vi "Controller 2.vi"(0 "Joystick Multiplier":dbl=1.0) -> (1 "Axes":T1, 2 "Buttons":T2)   [LabVIEW 2013]
uses:
  <vilib>/Rock Robotics/WPI/Joystick/WPI_JoystickGetSetRefNum.vi
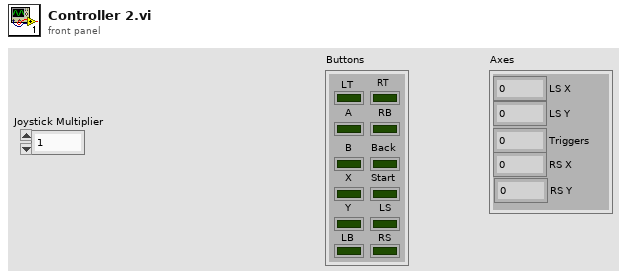
[diagram p1: front panel]
types:
  T1 = cluster{"LS X":dbl, "LS Y":dbl, "Triggers":dbl, "RS X":dbl, "RS Y":dbl}
  T2 = cluster{"LT":bool, "RT":bool, "A":bool, "B":bool, "X":bool, "Y":bool, "LB":bool, "RB":bool, "Back":bool, "Start":bool, "LS":bool, "RS":bool}
  T3 = typedef "WPI_JoystickDevRef.ctl" = cluster{"Device":T4}
  T4 = typedef "WPI_JoystickDeviceEnum.ctl" = enum16{"USB 1", "USB 2", "USB 3", "USB 4", "Kinect 1", "Kinect 2"}
  T5 = typedef "WPI_JoystickButtonState.ctl" = cluster{"Button 1":bool, "Button 2":bool, "Button 3":bool, "Button 4":bool, "Button 5":bool, "Button 6":bool, "Button 7":bool, "Button 8":bool, "Button 9":bool, "Button 10":bool, "Button 11":bool, "Button 12":bool}
  T6 = cluster{"axis 1 (x)":dbl, "axis 2 (y)":dbl, "axis 3 (throttle)":dbl, "axis 4":dbl, "axis 5":dbl, "axis 6":dbl}
  T7 = cluster{"axis 1 (x)":dbl, "axis 2 (y)":dbl, "axis 3 (throttle)":dbl, "axis 4":dbl, "axis 5":dbl}
  T8 = cluster{bool, bool, "Button 1":bool, "Button 2":bool, "Button 3":bool, "Button 4":bool, "Button 5":bool, "Button 6":bool, "Button 7":bool, "Button 8":bool, "Button 9":bool, "Button 10":bool}
  T9 = cluster{"[0]":dbl, "[1]":dbl, "[2]":dbl, "[3]":dbl, "[4]":dbl}
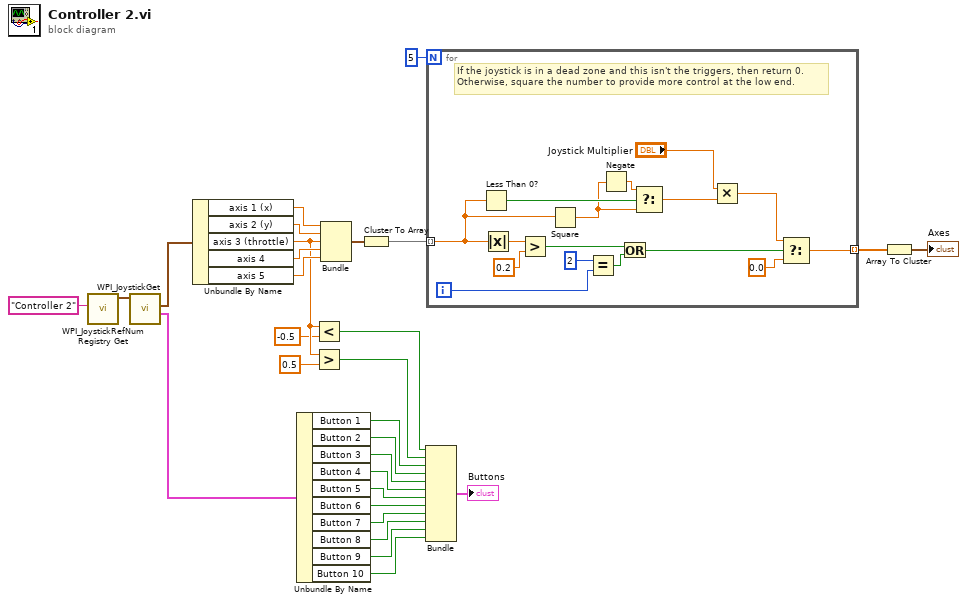
[diagram p0: block diagram]
diagram:
  n1 = call <vilib>:"WPI_JoystickRefNum Registry Get.vi"("refnum name"="Controller 2") -> ("JoystickDevRef"=w29:T3)  [unwired: 9 in, 1 out]
  n2 = call <vilib>:"WPI_JoystickGet.vi"("JoystickDevRef"=w29) -> ("Buttons"=w28:T5, "Axes"=w17:T6)  [unwired: 4 in, 1 out]
  n3 = Unbundle By Name(w17) -> ("axis 1 (x)"=w16:dbl, "axis 2 (y)"=w15:dbl, "axis 3 (throttle)"=w5:dbl, "axis 4"=w14:dbl, "axis 5"=w13:dbl)
  n4 = Unbundle By Name(w28) -> ("Button 1"=w27:bool, "Button 2"=w26:bool, "Button 3"=w25:bool, "Button 4"=w24:bool, "Button 5"=w23:bool, "Button 6"=w22:bool, "Button 7"=w21:bool, "Button 8"=w20:bool, "Button 9"=w19:bool, "Button 10"=w18:bool)
  n5 = Less?(x=w5, y=-0.5) -> (x < y?=w6:bool)
  n6 = Greater?(x=w5, y=0.5) -> (0:w2:bool)
  n7 = Bundle("axis 1 (x)"=w16, "axis 2 (y)"=w15, "axis 3 (throttle)"=w5, "axis 4"=w14, "axis 5"=w13) -> (w11:T7)  [unwired: 1 in]
  n8 = Cluster To Array(cluster=w11) -> (array=w9:dbl[])
  n9 = Bundle(w6, w2, "Button 1"=w27, "Button 2"=w26, "Button 3"=w25, "Button 4"=w24, "Button 5"=w23, "Button 6"=w22, "Button 7"=w21, "Button 8"=w20, "Button 9"=w19, "Button 10"=w18) -> (→"Buttons":T8)  [unwired: 1 in]
  n10 = for {
    N: 5 -> [_]
    tunnel: w9 -> [w40] mode=indexing
    tunnel: [w43] -> w8 mode=indexing
    i -> [w34]
    # "If the joystick is in a dead zone and this isn't the triggers, then return 0.\nOtherwise, square the number to provide more control at the low end."
    n11 = Less Than 0?(x=w40) -> (x < 0?=w41:bool)
    n12 = Absolute Value(x=w40) -> (abs(x)=w42:dbl)
    n13 = Greater?(x=w42, y=0.2) -> (0:w37:bool)
    n14 = Square(x=w40) -> (x^2=w39:dbl)
    n15 = Equal?(x=2, y=w34) -> (x = y?=w35:bool)
    n16 = Negate(x=w39) -> (-x=w38:dbl)
    n17 = Or(x=w37, y=w35) -> (x .or. y?=w36:bool)
    n18 = Select(t=w38, s=w41, f=w39) -> (s? t:f=w31:dbl)
    n19 = Multiply(x="Joystick Multiplier", y=w31) -> (x*y=w32:dbl)
    n20 = Select(t=w32, s=w36, f=0.0) -> (s? t:f=w43:dbl)
  }
  n21 = Array To Cluster(array=w8) -> (cluster=→"Axes":T9)
